vi "辅助定量定性分析结果显示表子VI.vi"(6 "疑似分层类缺陷数":dbl, 8 "疏松类缺陷数":dbl, 9 "其它缺陷数":dbl, 10 "总缺陷数":dbl, 11 "评定结果":dbl[][](array[numeric])) -> ()   [LabVIEW 2022 SP3]
panel:
  out "其它不明显缺陷个数":dbl
  out "疑似分层类缺陷个数":dbl
  out "疏松类缺陷个数":dbl
  out "总缺陷个数":dbl
  in  "退出":bool
  out "评定结果显示表":dbl[][](array[numeric])
  # "辅助定量定性分析结果显示表"
  # "缺陷编号"
  # "缺陷位置_X"
  # "缺陷位置_Y"
  # "缺陷长度(mm)"
  # "缺陷宽度(mm)"
  # "最大灰度值"
  # "最小灰度值"
  # "缺陷面积（mm2）"
  # "缺陷Z值（mm）"
  # "缺陷部位"
  # "缺陷性质"
  # "备注：\n（1）缺陷部位：0—蒙皮部位、1—筋条部位；\n（2）缺陷性质：1—疏松类缺陷、2—疑似分层类缺陷、0—其它轻微缺陷。"
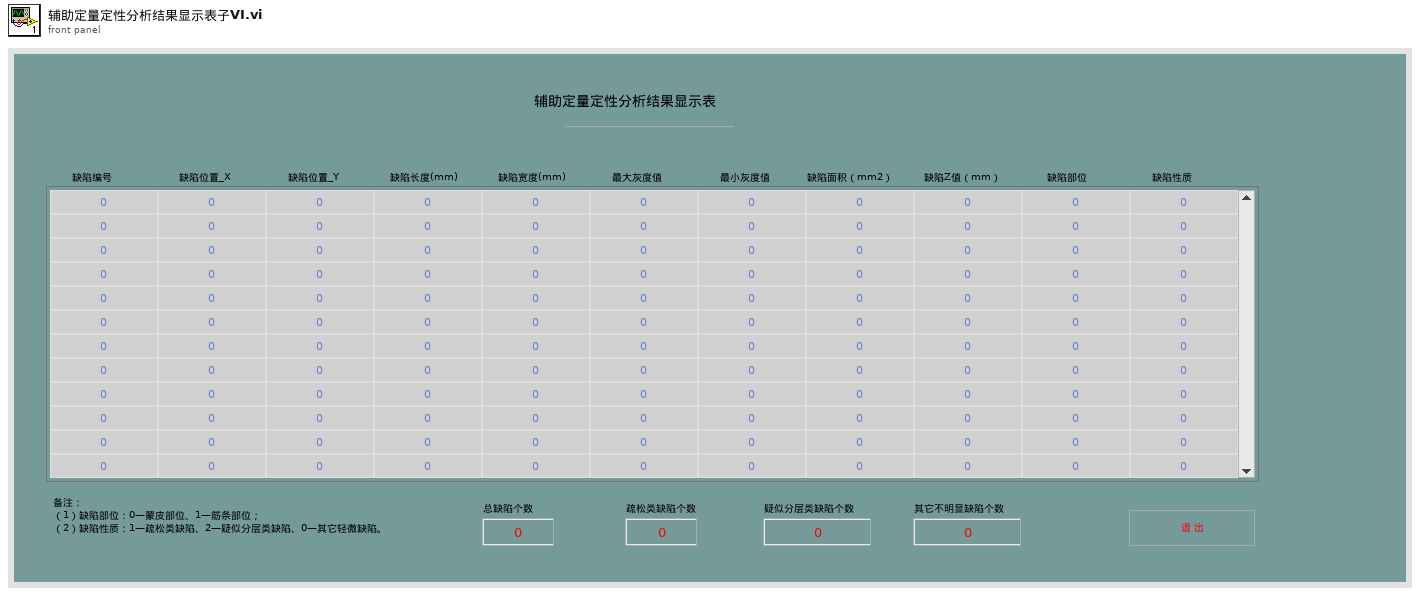
[diagram p1: front panel]
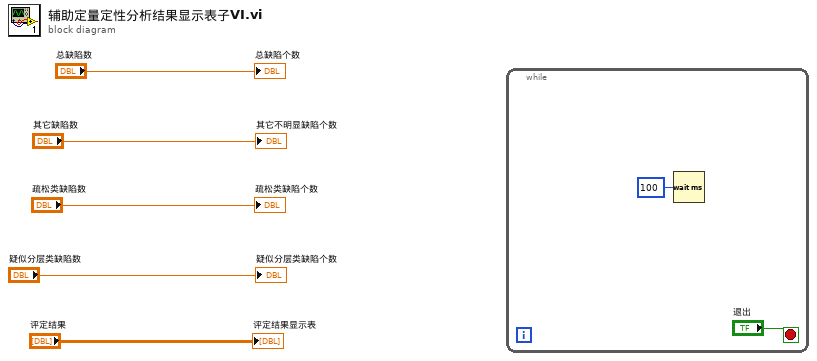
[diagram p0: block diagram]
diagram:
  n1 = while {
    stop <- "退出" stop-if-true
    n2 = Wait (ms)(milliseconds to wait=u32 100 ("等待时间（毫秒）")) -> ()  [unwired: 1 out]
  }
  "评定结果显示表" <- "评定结果"
  "其它不明显缺陷个数" <- "其它缺陷数"
  "疑似分层类缺陷个数" <- "疑似分层类缺陷数"
  "总缺陷个数" <- "总缺陷数"
  "疏松类缺陷个数" <- "疏松类缺陷数"
